vi "Create DAQ tasks--GUI.vi"(8 "error in (no error)":errorcluster, 10 "Device name":string, 11 "DAQ mod ID":i32) -> (0 "error out":errorcluster)   [LabVIEW 2020, in "GUI.lvlib"]
uses:
  GUI.lvlib
  NI DAQ/NI DAQ.lvlib
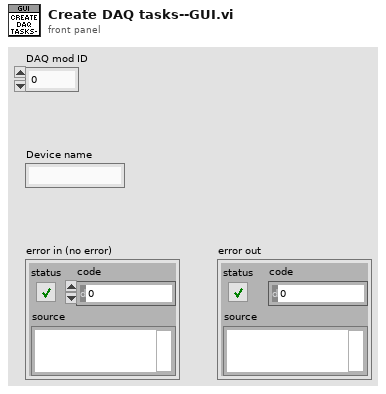
[diagram p1: front panel]
types:
  T1 = cluster{"input terminal configuration":i32, "minimum value":dbl, "maximum value":dbl}
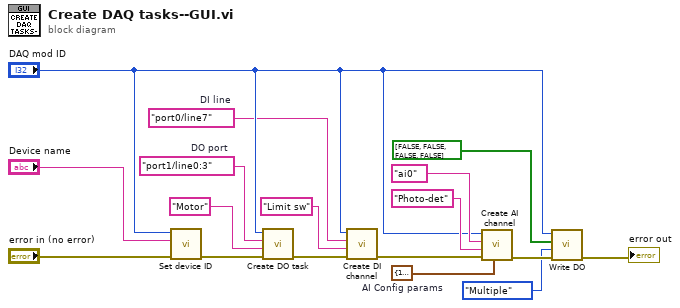
[diagram p0: block diagram]
diagram:
  w17 = T1 {"input terminal configuration"=10083, "minimum value"=0.0, "maximum value"=5.0}  # AI Config params
  w8 = tag "port0/line7"  # DI line
  w4 = tag "port1/line0:3"  # DO port
  n1 = call "Set device ID.vi"("error in"="error in (no error)", "Device ID"="Device name", "Module ID"="DAQ mod ID") -> ("error out"=w2:errorcluster)  [unwired: 8 in]
  n2 = call "Create DO task.vi"("error in"=w2, "Channel name"="Motor" ("Task name"), "lines"=w4, "Module ID"="DAQ mod ID") -> ("error out"=w6:errorcluster)  [unwired: 5 in, 2 out]
  n3 = call "Create DI channel.vi"("error in"=w6, "Channel name"="Limit sw", "Physical channel"=w8, "Module ID"="DAQ mod ID") -> ("error out"=w12:errorcluster)  [unwired: 7 in]
  n4 = call "Create AI channel.vi"("Config params"=w17, "error in"=w12, "Channel name"="Photo-det", "Physical channel"="ai0", "Module ID"="DAQ mod ID") -> ("error out"=w13:errorcluster)  [unwired: 6 in]
  n5 = call "Write DO.vi"("error in"=w13, "Samples"=enum16{"Single", "Multiple"}."Multiple", "Data"=bool[] [FALSE, FALSE, FALSE, FALSE], "Module ID"="DAQ mod ID") -> ("error out"=→"error out":errorcluster)  [unwired: 7 in]
